vi "Get information from table.vi"(4 "Numeric":i32, 6 "Table":string[][](array[string])) -> (1 "Average/Samples":string, 2 "N Sample":string, 3 "Offset":string, 5 "Mul.Factor":string, 7 "Units":string, 9 "Test Name":string, 10 "Request Value":string, 11 "Accurrance":string)   [LabVIEW 2017]
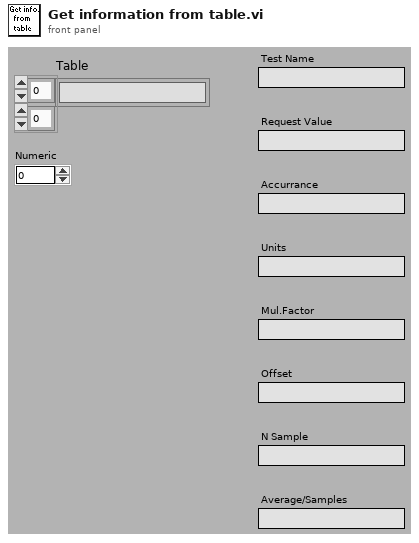
[diagram p1: front panel]
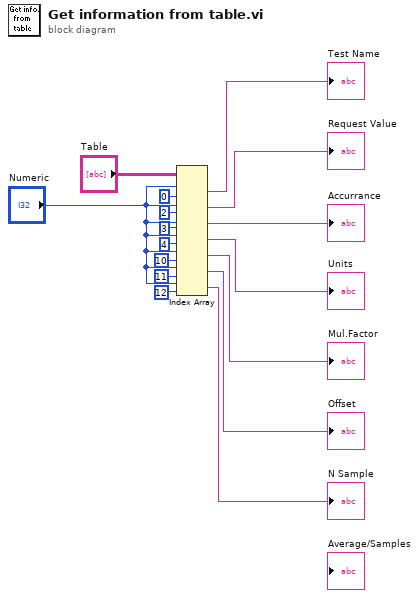
[diagram p0: block diagram]
diagram:
  n1 = Index Array(array="Table", index (row) #1="Numeric", index (col) #1=0 ("disabled index (col)"), index (row) #2="Numeric", index (col) #2=2 ("disabled index (col)"), index (row) #3="Numeric", index (col) #3=3 ("disabled index (col)"), index (row) #4="Numeric", index (col) #4=4 ("disabled index (col)"), index (row) #5="Numeric", index (col) #5=10 ("disabled index (col)"), index (row) #6="Numeric", index (col) #6=11 ("disabled index (col)"), index (row) #7="Numeric", index (col) #7=12 ("disabled index (col)")) -> (element #1=→"Test Name":string, element #2=→"Request Value":string, element #3=→"Accurrance":string, element #4=→"Units":string, element #5=→"Mul.Factor":string, element #6=→"Offset":string, element #7=→"N Sample":string)
